vi "CS++Main-Linux.vi"() -> ()   [LabVIEW 2016]
doc: "This VI illustrates how to use the <b>Launch CS++StartActor.vi</b> as subVI.\n\nYou may create a copy and add your project specific stuff."
uses:
  Packages/CSPP_Core/Actors/CS++StartActor/CS++StartActor.lvlib
panel:
  out "Attributes found?":bool
  out "Error Out":errorcluster
  in  "Error In":errorcluster
  in  "CS++Factory":path
  in  "Start Actor":string="CS++StartActor"
  in  "DB Connection String":string
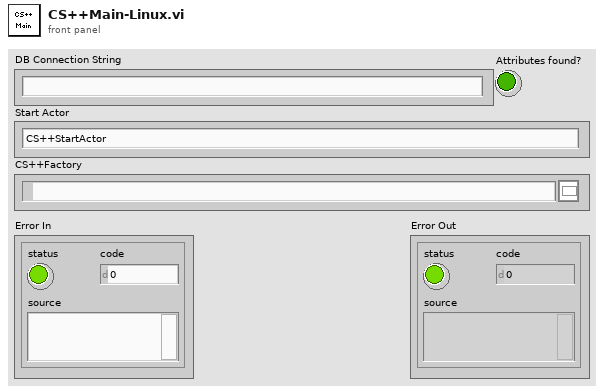
[diagram p1: front panel]
types:
  T1 = cluster{"Classname":string, "CS++Messages":refnum<class "Message.lvclass">[]}[]
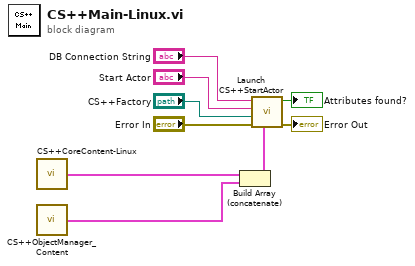
[diagram p0: block diagram]
diagram:
  n1 = call "CS++CoreContent-Linux.vi"() -> ("CS++Classes & Messages"=w1:T1)  [unwired: 1 in]
  n2 = call "CS++ObjectManager_Content.vi"() -> ("CS++Classes & Messages"=w3:T1)  [unwired: 1 in]
  n3 = Build Array (concatenate)(w1, w3) -> (w2:T1)
  n4 = call "Launch CS++StartActor.vi"("CS++Classes & Messages"=w2, "Error In"="Error In", "CS++Factory"="CS++Factory", "Start Actor"="Start Actor", "DB Connection String"="DB Connection String") -> ("Error Out"=→"Error Out":errorcluster, "Attributes found?"=→"Attributes found?":bool)  [unwired: 4 in, 1 out]
